vi "JLINKARM DecodeHexStr.vi"(8 "错误输入（无错误）":errorcluster, 11 "HexStr":string) -> (0 "错误输出":errorcluster, 3 "LineHexData":T1 {"CRC" format="%02x"; "Data" format="%02x"; "Addr" format="%04x"; "Len" format="%02x"})   [LabVIEW 2016]
uses:
  <userlib>/LV-JLinkARM/App/JLinkARM LineHexDataType.ctl
  <userlib>/LV-JLinkARM/App/JLINKARM DataType.ctl
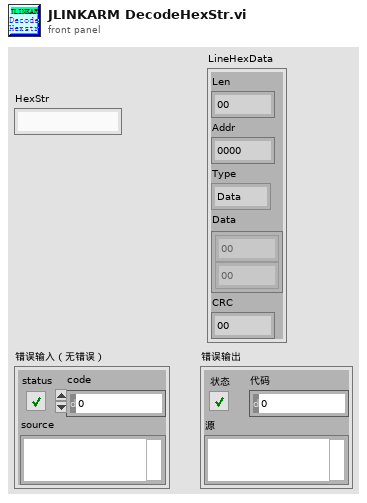
[diagram p1: front panel]
types:
  T1 = typedef "JLinkARM LineHexDataType.ctl" = cluster{"Len":u8, "Addr":u16, "Type":T2, "Data":u8[], "CRC":u8}
  T2 = typedef "JLINKARM DataType.ctl" = enum16{"Data", "EndofFile", "ExtSegAdd", "StartSegAddr", "ExtLinearAddr", "StartLinearAddr"}
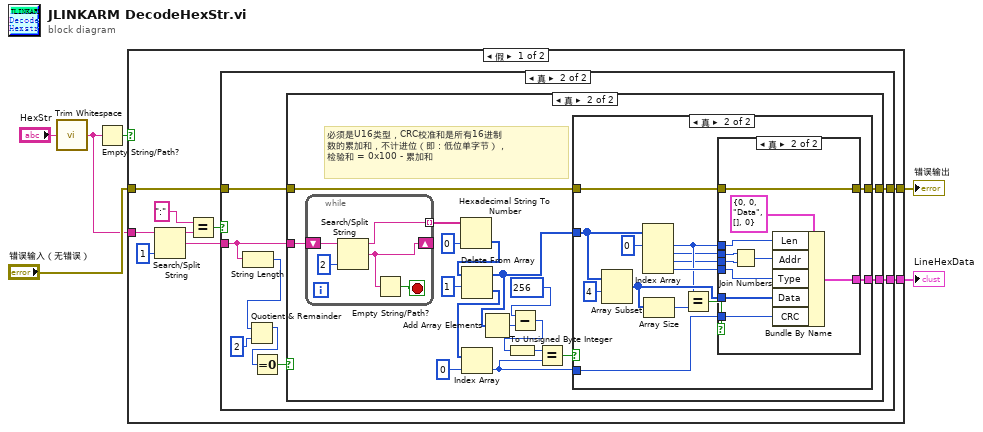
[diagram p0: block diagram]
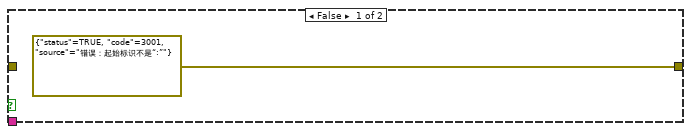
[diagram p2: hidden frame]
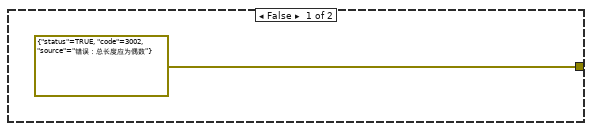
[diagram p3: hidden frame]
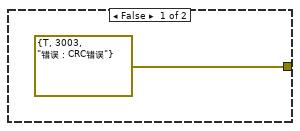
[diagram p4: hidden frame]
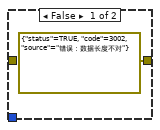
[diagram p5: hidden frame]
diagram:
  n1 = call <vilib>:"Trim Whitespace.vi"("string"="HexStr") -> ("trimmed string"=w1:string)  [unwired: 1 in]
  n2 = Empty String/Path?(string/path=w1) -> (empty?=w2:bool)
  n3 = case shown="假" w2 {
    tunnel: "错误输入（无错误）" -> [w15 w74]
    tunnel: [w14 w74] -> w5
    tunnel: [w13 _] -> w4
    tunnel: w1 -> [w7 _]
    frame False {
      n4 = Search/Split String(string=w7, offset (0)=1 ("偏移量(0)")) -> (substring before match=w10:string, match + rest of string=w8:string)  [unwired: 1 in, 1 out]
      n5 = Equal?(x=":", y=w10) -> (x = y?=w12:bool)
      n6 = case shown="真" w12 {
        tunnel: w8 -> [_ w24]
        tunnel: [_ w19] -> w13
        tunnel: [errorcluster {"status"=TRUE, "code"=3001, "source"="错误：起始标识不是“:”"} ("error out") w18] -> w14
        tunnel: w15 -> [_ w17]
        frame False {
        }
        frame True {
          n7 = String Length(string=w24) -> (length=w23:i32)
          n8 = Quotient & Remainder(x=w23, y=2) -> (x-y*floor(x/y)=w21:i32)  [unwired: 1 out]
          n9 = Equal To 0?(x=w21) -> (x = 0?=w20:bool)
          n10 = case shown="真" w20 {
            tunnel: w24 -> [_ w41]
            tunnel: [_ w30] -> w19
            tunnel: [errorcluster {"status"=TRUE, "code"=3002, "source"="错误：总长度应为偶数"} ("error out") w29] -> w18
            tunnel: w17 -> [_ w28]
            frame False {
            }
            frame True {
              # "必须是U16类型，CRC校准和是所有16进制\n数的累加和，不计进位（即：低位单字节），\n检验和 = 0x100 - 累加和"
              n11 = while {
                shift-right: [w70] -> _
                shift-left: w41 -> [w73]
                tunnel: [w71] -> w42 mode=indexing
                stop <- w69 stop-if-true
                n12 = Search/Split String(string=w73, offset (0)=2 ("偏移量(0)")) -> (substring before match=w71:string, match + rest of string=w70:string)  [unwired: 1 in, 1 out]
                n13 = Empty String/Path?(string/path=w70) -> (empty?=w69:bool)
              }
              n14 = Hexadecimal String To Number(string=w42, default (0uL)=u16 0 ("默认(0 U32)")) -> (number=w38:u16[])  [unwired: 1 in, 1 out]
              n15 = Delete From Array(array=w38, length=1 ("长度")) -> (deleted portion=w34:u16[], array with subset deleted=w36:u16[])  [unwired: 1 in]
              n16 = Index Array(array=w34, index=0 ("索引")) -> (element=w32:u16)
              n17 = Add Array Elements(numeric array=w36) -> (sum=w35:u16)
              n18 = Subtract(x=u32 256, y=w35) -> (x-y=w27:u32)
              n19 = To Unsigned Byte Integer(number=w27) -> (unsigned 8bit integer=w26:u8)
              n20 = Equal?(x=w26, y=w32) -> (x = y?=w31:bool)
              n21 = case shown="真" w31 {
                tunnel: w36 -> [_ w53]
                tunnel: w32 -> [_ w54]
                tunnel: [_ w48] -> w30
                tunnel: [errorcluster {"status"=TRUE, "code"=3003, "source"="错误：CRC错误"} ("error out") w47] -> w29
                tunnel: w28 -> [_ w46]
                frame False {
                }
                frame True {
                  n22 = Array Subset(array=w53, index=4 ("索引")) -> (w52:u16[])  [unwired: 1 in]
                  n23 = Index Array(array=w53, index #1=0 ("索引")) -> (element #1=w50:u16, element #2=w45:u16, element #3=w44:u16, element #4=w56:u16)  [unwired: 3 in]
                  n24 = Array Size(array=w52) -> (size(s)=w51:i32)
                  n25 = Equal?(x=w50, y=w51) -> (x = y?=w49:bool)
                  n26 = case shown="真" w49 {
                    tunnel: w45 -> [_ w67]
                    tunnel: w44 -> [_ w66]
                    tunnel: w56 -> [_ w64]
                    tunnel: w54 -> [_ w63]
                    tunnel: w52 -> [_ w62]
                    tunnel: w50 -> [_ w61]
                    tunnel: [_ w60] -> w48
                    tunnel: [errorcluster {"status"=TRUE, "code"=3002, "source"="错误：数据长度不对"} ("error out") w59] -> w47
                    tunnel: w46 -> [_ w59]
                    frame False {
                    }
                    frame True {
                      n27 = Join Numbers(hi=w67, lo=w66) -> ((hi.lo)=w65:u32)
                      n28 = Bundle By Name(cluster=T1 {"Len"=0, "Addr"=0, "Type"=enum."Data", "Data"=[], "CRC"=0} ("LineHexData"), "Len"=w61, "Addr"=w65, "Type"=w64, "Data"=w62, "CRC"=w63) -> (w60:T1)
                    }
                  }
                }
              }
            }
          }
        }
      }
    }
    frame True {
    }
  }
  "错误输出" <- w5
  "LineHexData" <- w4
